vi "高锰酸钾-ORP滴定曲线(子VI).vi"   [LabVIEW 2016, in "斯坦道CODMn.lvlib"]
uses:
  <vilib>/ptbypt/NI_PtbyPt.lvlib
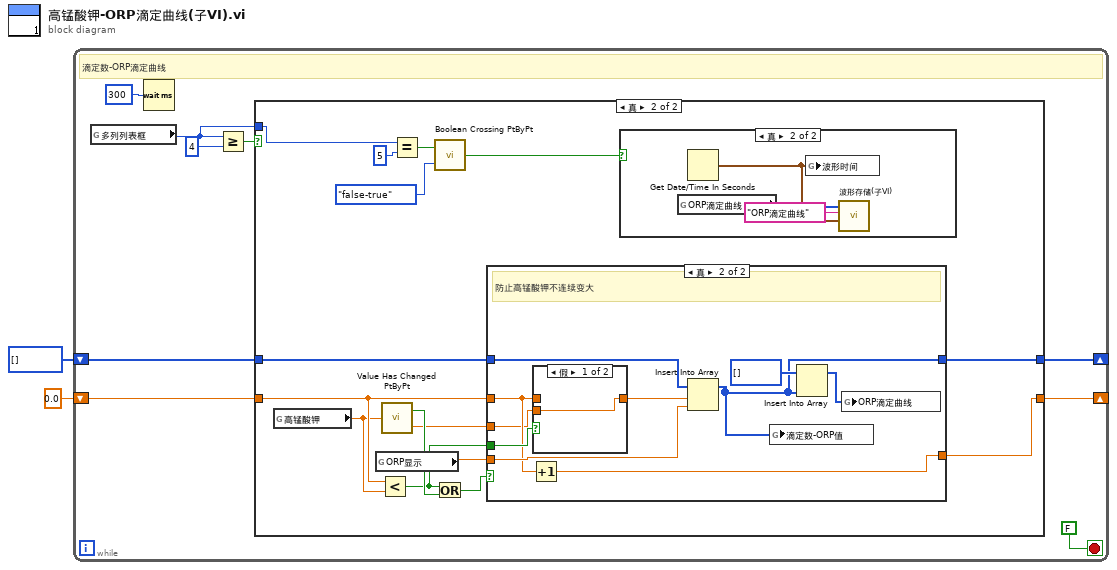
[diagram p0: block diagram]
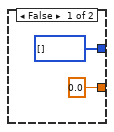
[diagram p2: hidden frame]
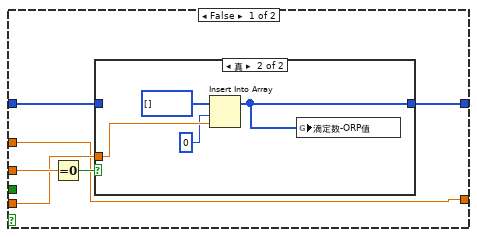
[diagram p4: hidden frame]
diagram:
  n1 = while {
    shift-right: [w8] -> _
    shift-left: u16[] [] ("ORP滴定曲线") -> [w9]
    shift-right: [w4] -> _
    shift-left: 0.0 -> [w5]
    stop <- FALSE stop-if-true
    # "滴定数-ORP滴定曲线"
    n2 = global read "运行时序全局变量.vi" "多列列表框"() -> (w3:i32)
    n3 = Wait (ms)(milliseconds to wait=u32 300 ("等待时间（毫秒）")) -> ()  [unwired: 1 out]
    n4 = Greater Or Equal?(x=w3, y=4) -> (x >= y?=w6:bool)
    n5 = case shown="真" w6 {
      tunnel: w9 -> [_ w28]
      tunnel: [u16[] [] ("ORP滴定曲线") w27] -> w8
      tunnel: w5 -> [_ w19]
      tunnel: [0.0 w18] -> w4
      tunnel: w3 -> [_ w16]
      frame False {
      }
      frame True {
        n6 = global read "COD内部交互全局.vi" "高锰酸钾"() -> (w15:dbl)
        n7 = global read "COD内部交互全局.vi" "ORP显示"() -> (w14:dbl)
        n8 = Less?(x=w19, y=w15) -> (x < y?=w17:bool)
        n9 = call <vilib>:"Value Has Changed PtByPt.vi"("input data point"=w15) -> ("has changed"=w26:bool, "output data point"=w25:dbl)  [unwired: 1 in]
        n10 = Equal?(x=w16, y=5) -> (x = y?=w23:bool)
        n11 = call <vilib>:"Boolean Crossing PtByPt.vi"("direction"=enum16{"either", "false-true", "true-false"}."false-true", "input"=w23) -> ("crossing"=w21:bool)  [unwired: 1 in]
        n12 = Or(x=w17, y=w26) -> (x .or. y?=w20:bool)
        n13 = case shown="真" w20 {
          tunnel: w28 -> [w36 w51]
          tunnel: [w35 w43] -> w27
          tunnel: w25 -> [w37 w45]
          tunnel: w14 -> [w33 w50]
          tunnel: w19 -> [w32 w47]
          tunnel: [w32 w49] -> w18
          tunnel: w17 -> [_ w48]
          frame False {
            n14 = Equal To 0?(x=w37) -> (x = 0?=w34:bool)
            n15 = case shown="真" w34 {
              tunnel: [w38 w39] -> w35
              tunnel: w36 -> [w38 _]
              tunnel: w33 -> [_ w41]
              frame False {
              }
              frame True {
                n16 = Insert Into Array(array=u16[] [] ("ORP滴定曲线"), index=0 ("索引"), new element=w41) -> (w39:u16[])
                n17 = global write "COD内部交互全局.vi" "滴定数-ORP值"(w39) -> ()
              }
            }
          }
          frame True {
            # "防止高锰酸钾不连续变大"
            n18 = Increment(x=w47) -> (x+1=w49:dbl)
            n19 = case shown="假" w48 {
              tunnel: w47 -> [_ w54]
              tunnel: [w53 w54] -> w46
              tunnel: w45 -> [w53 _]
              frame False {
              }
              frame True {
              }
            }
            n20 = Insert Into Array(array=w51, index=w46, new element=w50) -> (w43:u16[])
            n21 = global write "COD内部交互全局.vi" "滴定数-ORP值"(w43) -> ()
            n22 = Insert Into Array(array=u16[] [] ("ORP滴定曲线"), new element=w43) -> (w44:u16[])  [unwired: 1 in]
            n23 = global write "COD内部交互全局.vi" "ORP滴定曲线"(w44) -> ()
          }
        }
        n24 = case shown="真" w21 {
          frame False {
          }
          frame True {
            n25 = global read "COD内部交互全局.vi" "ORP滴定曲线"() -> (w31:u16[])
            n26 = Get Date/Time In Seconds() -> (seconds since 1Jan1904=w30:timestamp)
            n27 = global write "COD内部交互全局.vi" "波形时间"(w30) -> ()
            n28 = call "波形存储(子VI).vi"("波形时间"=w30, "condition"="ORP滴定曲线", "ORP滴定曲线"=w31) -> ()  [unwired: 9 in]
          }
        }
      }
    }
  }
